vi "Scrittura file.vi"(5 "Mean Array":dbl[](array[numeric]) format="%0.2f", 6 "Frequency":dbl, 7 "Dev. Array":dbl[](array[numeric]) format="%0.2f", 8 "error in (no error)":errorcluster, 9 "Load":dbl, 10 "Voltage":dbl, 11 "Byte Stream File in":refnum<file>) -> (0 "error out":errorcluster, 3 "Byte Stream File out":refnum<file>)   [LabVIEW 2018]
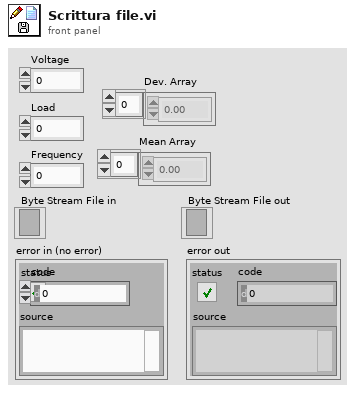
[diagram p1: front panel]
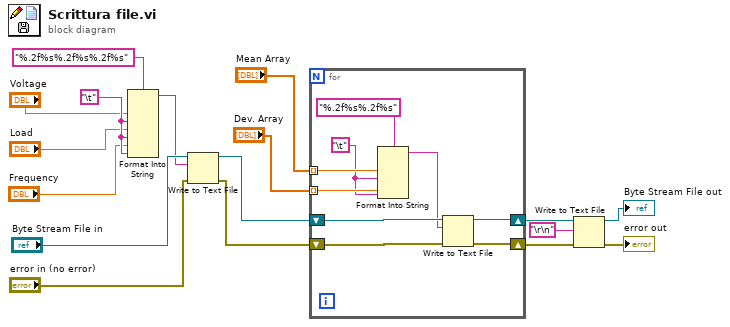
[diagram p0: block diagram]
diagram:
  w6 = "\t"
  n1 = Format Into String(format string="%.2f%s%.2f%s%.2f%s", "Voltage", w6, "Load", w6, "Frequency", w6) -> (resulting string=w13:string)  [unwired: 2 in, 1 out]
  n2 = Write to Text File(file (use dialog)="Byte Stream File in", text=w13, error in="error in (no error)") -> (refnum out=w15:refnum<file>, error out=w14:errorcluster)  [unwired: 1 in, 1 out]
  n3 = for {
    shift-right: [w26] -> w10
    shift-left: w14 -> [w24]
    shift-right: [w25] -> w9
    shift-left: w15 -> [w23]
    tunnel: "Dev. Array" -> [w21] mode=indexing
    tunnel: "Mean Array" -> [w20] mode=indexing
    w19 = "\t"
    n4 = Format Into String(format string="%.2f%s%.2f%s", w20, w19, w21, w19) -> (resulting string=w18:string)  [unwired: 2 in, 1 out]
    n5 = Write to Text File(file (use dialog)=w23, text=w18, error in=w24) -> (refnum out=w25:refnum<file>, error out=w26:errorcluster)  [unwired: 1 in, 1 out]
  }
  n6 = Write to Text File(file (use dialog)=w9, text="\r\n", error in=w10) -> (refnum out=→"Byte Stream File out":refnum<file>, error out=→"error out":errorcluster)  [unwired: 1 in, 1 out]
